vi "SaveAsFileDialog.vi"(8 "error in":errorcluster, 11 "Current File":path) -> (0 "error out":errorcluster, 1 "Cancelled?":bool, 2 "selected file path":path caption="selected path", 3 "Current File out":path)   [LabVIEW 2018, in "Test.lvclass"]
uses:
  Test.lvclass
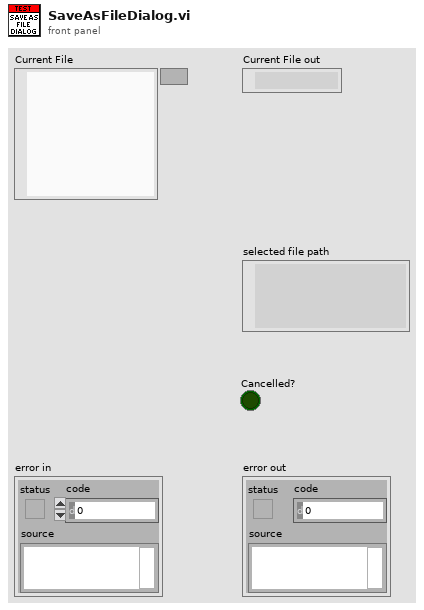
[diagram p1: front panel]
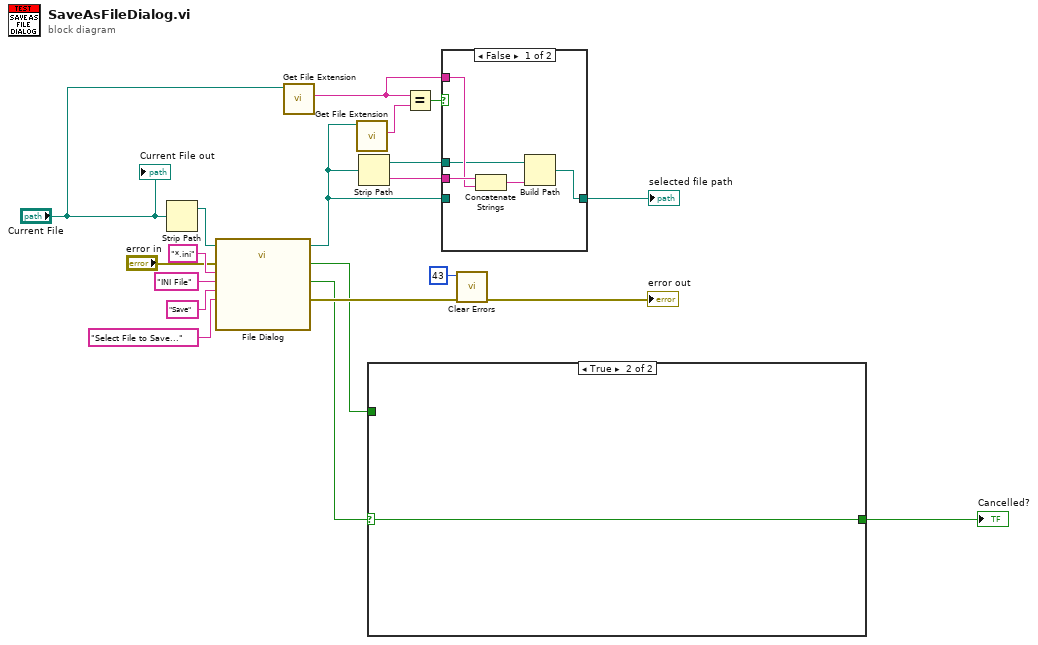
[diagram p0: block diagram]
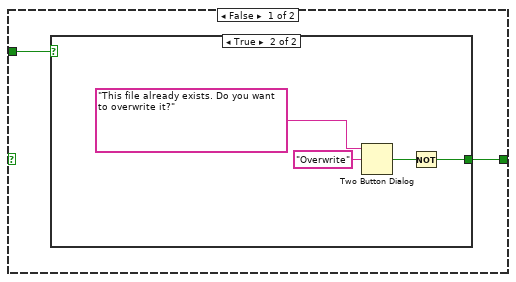
[diagram p3: hidden frame]
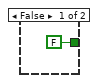
[diagram p4: hidden frame]
diagram:
  n1 = Strip Path(path="Current File") -> (stripped path=w16:path)  [unwired: 1 out]
  n2 = call "File Dialog"("start path"=w16, "prompt"="Select File to Save...", "button label"="Save", "error in"="error in", "pattern (all files)"="*.ini", "pattern label"="INI File") -> ("selected path"=w5:path, "exists"=w13:bool, "cancelled"=w12:bool, "error out"=w14:errorcluster)  [unwired: 6 in]
  n3 = call <vilib>:"Get File Extension.vi"("file"="Current File") -> ("lowercase file extension"=w2:string)  [unwired: 6 in, 4 out]
  n4 = call <vilib>:"Get File Extension.vi"("file"=w5) -> ("lowercase file extension"=w7:string)  [unwired: 6 in, 4 out]
  n5 = Strip Path(path=w5) -> (stripped path=w1:path, name=w3:string)
  n6 = case shown="True" w12 {
    selector: w12 -> [_ w28]
    tunnel: w13 -> [w22 _]
    tunnel: [w21 w28] -> w11
    frame False {
      n7 = case shown="True" w22 {
        tunnel: [FALSE w24] -> w21
        frame False {
        }
        frame True {
          n8 = Two Button Dialog(message="This file already exists. Do you want to overwrite it?", 2:"Overwrite" ("T button name (\"OK\")")) -> (T button?=w25:bool)  [unwired: 1 in]
          n9 = Not(x=w25) -> (.not. x?=w24:bool)
        }
      }
    }
    frame True {
    }
  }
  "Cancelled?" <- w11
  n10 = Equal?(x=w2, y=w7) -> (x = y?=w6:bool)
  n11 = case shown="False" w6 {
    tunnel: w5 -> [_ w34]
    tunnel: [w29 w34] -> w4
    tunnel: w3 -> [w33 _]
    tunnel: w2 -> [w32 _]
    tunnel: w1 -> [w30 _]
    frame False {
      n12 = Concatenate Strings(w33, w32) -> (w31:string)
      n13 = Build Path(base path=w30, name or relative path=w31) -> (appended path=w29:path)
    }
    frame True {
    }
  }
  "selected file path" <- w4
  n14 = call <vilib>:"Clear Errors.vi"("error in (no error)"=w14, "specific error code to clear (0: all)"=43) -> ("error out"=→"error out":errorcluster)  [unwired: 4 in, 1 out]
  "Current File out" <- "Current File"
